vi "Create Case Description.vi"(10 "Case":string, 11 "Test Result Tree V2 in":refnum<class "Test Result Tree V2.lvclass">) -> (2 "Description":string, 3 "Test Result Tree V2 in 2":refnum<class "Test Result Tree V2.lvclass">)   [LabVIEW 2020, in "Test Result Tree V2.lvclass"]
uses:
  Test Result Tree V2.lvclass
  Result/Status.ctl
  Test Result Tree Test/Private/Counter Map Key.ctl
  Test Result Tree V2.lvclass/Test Result Tree V2.ctl
  Result/Result.lvlib
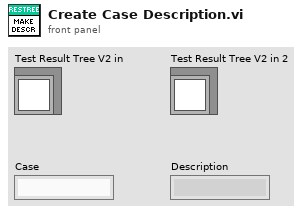
[diagram p1: front panel]
types:
  T1 = typedef "Result.lvlib/Status.ctl" = enum16{"", "Passed", "Failed", "Error", "Skipped", "Setup Error", "Broken", "Teardown Error"}
  T2 = typedef "Test Result Tree V2.lvclass/Counter Map Key.ctl" = cluster{"Test Case":string, "Status":T1}
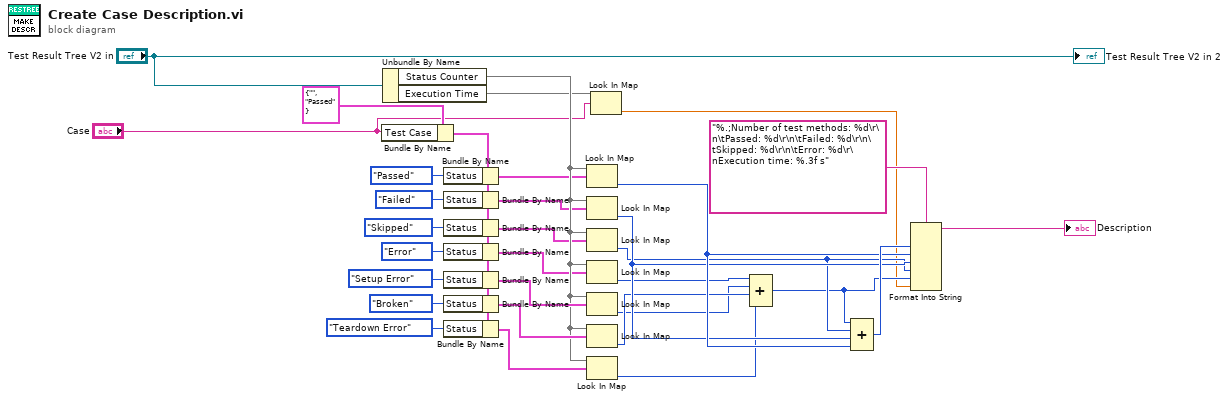
[diagram p0: block diagram]
diagram:
  n1 = Bundle By Name(cluster=T2 {"Test Case"="", "Status"=enum."Passed"} ("key"), "Test Case"="Case") -> (w21:T2)
  n2 = Unbundle By Name("Test Result Tree V2 in") -> ("Status Counter"=w18:map{T2, i32}, "Execution Time"=w3:map{string, dbl})
  n3 = Bundle By Name(cluster=w21, "Status"=Status."Passed") -> (w6:T2)
  n4 = Bundle By Name(cluster=w21, "Status"=Status."Failed") -> (w9:T2)
  n5 = Bundle By Name(cluster=w21, "Status"=Status."Skipped") -> (w11:T2)
  n6 = Bundle By Name(cluster=w21, "Status"=Status."Error") -> (w12:T2)
  n7 = Bundle By Name(cluster=w21, "Status"=Status."Setup Error") -> (w19:T2)
  n8 = Bundle By Name(cluster=w21, "Status"=Status."Broken") -> (w20:T2)
  n9 = Bundle By Name(cluster=w21, "Status"=Status."Teardown Error") -> (w30:T2)
  n10 = Look In Map(map=w18, key=w6) -> (value=w28:i32)  [unwired: 1 in, 1 out]
  n11 = Look In Map(map=w18, key=w9) -> (value=w27:i32)  [unwired: 1 in, 1 out]
  n12 = Look In Map(map=w18, key=w11) -> (value=w26:i32)  [unwired: 1 in, 1 out]
  n13 = Look In Map(map=w18, key=w12) -> (value=w13:i32)  [unwired: 1 in, 1 out]
  n14 = Look In Map(map=w18, key=w19) -> (value=w22:i32)  [unwired: 1 in, 1 out]
  n15 = Look In Map(map=w18, key=w20) -> (value=w23:i32)  [unwired: 1 in, 1 out]
  n16 = Look In Map(map=w18, key=w30) -> (value=w24:i32)  [unwired: 1 in, 1 out]
  n17 = Look In Map(map=w3, key="Case") -> (value=w1:dbl)  [unwired: 1 in, 1 out]
  n18 = Compound Arithmetic op=ADD(w13, w22, w23, w24) -> (w25:i32)
  n19 = Compound Arithmetic op=ADD(w25, w26, w27, w28) -> (w29:i32)
  n20 = Format Into String(format string="%.;Number of test methods: %d\r\n\tPassed: %d\r\n\tFailed: %d\r\n\tSkipped: %d\r\n\tError: %d\r\nExecution time: %.3f s", w29, w28, w27, w26, w25, w1) -> (resulting string=→"Description":string)  [unwired: 2 in, 1 out]
  "Test Result Tree V2 in 2" <- "Test Result Tree V2 in"
